vi "Check Data Model.vi"(8 "error in (no error)":errorcluster, 11 "device data model in":refnum<class "ICPCON ET Data Model.lvclass">) -> (0 "error out":errorcluster, 3 "device data model out":refnum<class "ICPCON ET Data Model.lvclass">)   [LabVIEW 2021, in "ICPCON ET Data Model.lvclass"]
doc: "This VI ensures that the data model has at least 65,535 values of every type. This is required for certain modbus function codes."
uses:
  ICPCON ET Data Model.lvclass
  ICPCON ET Data Model.lvclass/ICPCON ET Data Model.ctl
  Type Definitions/Data Model.ctl
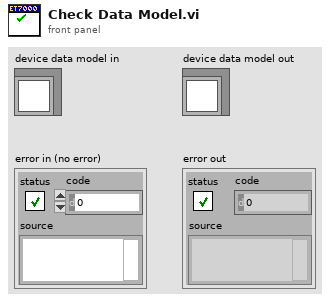
[diagram p1: front panel]
types:
  T1 = typedef "ICPCON ET Data Model.lvclass/Data Model.ctl" = cluster{"UTC":u64, "DI":bool[], "DO":bool[], "IR":u16[], "HR":u16[], "ES":u8}
  T2 = typedef "Device Data Model.lvclass/N channel.ctl" = cluster{"N DI channel":i32, "N DO channel":i32, "N AI channel":i32, "N AO channel":i32}
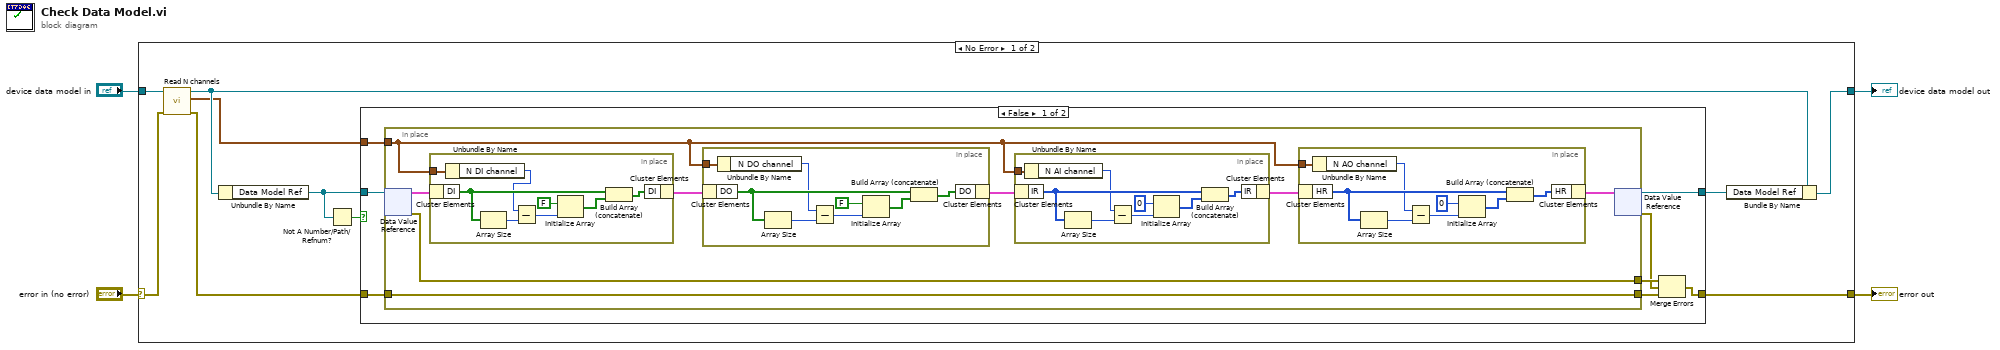
[diagram p0: block diagram]
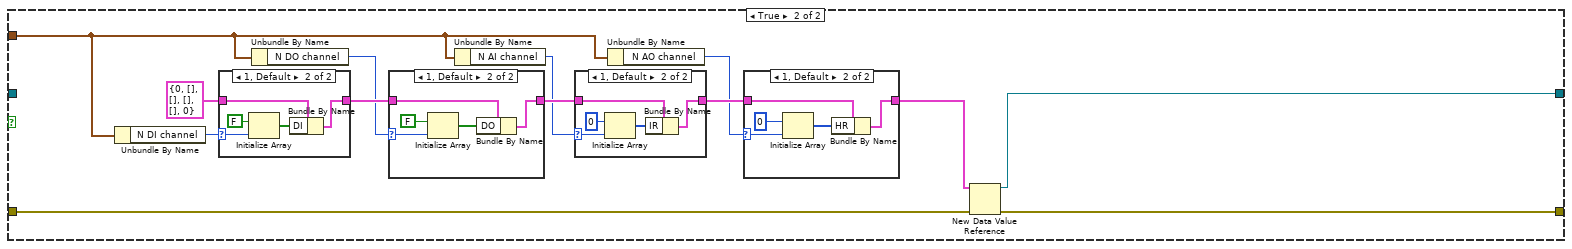
[diagram p2: hidden frame]
diagram:
  n1 = case shown="No Error" "error in (no error)" {
    selector: "error in (no error)" -> [w7 w101]
    tunnel: "device data model in" -> [w9 w100]
    tunnel: [w14 w100] -> w3
    tunnel: [w10 w101] -> w2
    frame No Error {
      n2 = call-dynamic "Read N channels.vi"("error in (no error)"=w7, "device data model in"=w9) -> ("error out"=w6:errorcluster, "N channel"=w5:T2, "device data model out"=w8:refnum<class "ICPCON ET Data Model.lvclass">)  [unwired: 7 in]
      n3 = Unbundle By Name(w8) -> ("Data Model Ref"=w12:refnum<data-value>)
      n4 = Not A Number/Path/Refnum?(number/path/refnum=w12) -> (NaN/Path/Refnum?=w11:bool)
      n5 = case shown="False" w11 {
        tunnel: w6 -> [w22 w75]
        tunnel: w12 -> [w21 _]
        tunnel: [w20 w73] -> w13
        tunnel: [w18 w74] -> w10
        tunnel: w5 -> [w15 w64]
        frame False {
          n6 = in-place {
            in-place-border: w22 -> [w24]
            in-place-border: [w25] -> w19
            in-place-border: [w24] -> w16
            in-place-border: w15 -> [w23]
            n7 = in-place-dvr #1(w21) -> (w30:T1, w25:errorcluster)
            n8 = in-place {
              in-place-border: w23 -> [w56]
              n9 = in-place-cluster #2(w30) -> ("DI"=w59:bool[])
              n10 = Unbundle By Name(w56) -> ("N DI channel"=w55:i32)
              n11 = Array Size(array=w59) -> (size(s)=w62:i32)
              n12 = Subtract(x=w55, y=w62) -> (x-y=w61:i32)
              n13 = Initialize Array(FALSE ("Boolean"), w61) -> (w60:bool[])
              n14 = Build Array (concatenate)(w59, w60) -> (w57:bool[])
              n15 = in-place-cluster #2("DI"=w57) -> (w29:T1)
            }
            n16 = in-place {
              in-place-border: w23 -> [w48]
              n17 = in-place-cluster #3(w29) -> ("DO"=w52:bool[])
              n18 = Unbundle By Name(w48) -> ("N DO channel"=w47:i32)
              n19 = Array Size(array=w52) -> (size(s)=w54:i32)
              n20 = Subtract(x=w47, y=w54) -> (x-y=w50:i32)
              n21 = Initialize Array(FALSE ("Boolean"), w50) -> (w53:bool[])
              n22 = Build Array (concatenate)(w52, w53) -> (w49:bool[])
              n23 = in-place-cluster #3("DO"=w49) -> (w27:T1)
            }
            n24 = in-place {
              in-place-border: w23 -> [w39]
              n25 = in-place-cluster #4(w27) -> ("IR"=w43:u16[])
              n26 = Unbundle By Name(w39) -> ("N AI channel"=w40:i32)
              n27 = Array Size(array=w43) -> (size(s)=w46:i32)
              n28 = Subtract(x=w40, y=w46) -> (x-y=w45:i32)
              n29 = Initialize Array(u16 0, w45) -> (w44:u16[])
              n30 = Build Array (concatenate)(w43, w44) -> (w42:u16[])
              n31 = in-place-cluster #4("IR"=w42) -> (w28:T1)
            }
            n32 = in-place {
              in-place-border: w23 -> [w32]
              n33 = in-place-cluster #5(w28) -> ("HR"=w36:u16[])
              n34 = Unbundle By Name(w32) -> ("N AO channel"=w31:i32)
              n35 = Array Size(array=w36) -> (size(s)=w38:i32)
              n36 = Subtract(x=w31, y=w38) -> (x-y=w35:i32)
              n37 = Initialize Array(u16 0, w35) -> (w37:u16[])
              n38 = Build Array (concatenate)(w36, w37) -> (w34:u16[])
              n39 = in-place-cluster #5("HR"=w34) -> (w26:T1)
            }
            n40 = in-place-dvr #1(w26) -> (w20:refnum<data-value>, w17:errorcluster)
          }
          n41 = Merge Errors(w19, w17, w16) -> (w18:errorcluster)
        }
        frame True {
          n42 = Unbundle By Name(w64) -> ("N DI channel"=w68:i32)
          n43 = case shown="1, Default" w68 {
            selector: w68 -> [_ w83]
            tunnel: T1 {"UTC"=0, "DI"=[], "DO"=[], "IR"=[], "HR"=[], "ES"=0} ("Data Model") -> [w82 w86]
            tunnel: [w82 w84] -> w72
            frame 0 {
            }
            frame 1, Default {
              n44 = Initialize Array(FALSE ("Boolean"), w83) -> (w85:bool[])
              n45 = Bundle By Name(cluster=w86, "DI"=w85) -> (w84:T1)
            }
          }
          n46 = Unbundle By Name(w64) -> ("N DO channel"=w67:i32)
          n47 = case shown="1, Default" w67 {
            selector: w67 -> [_ w78]
            tunnel: w72 -> [w76 w81]
            tunnel: [w76 w79] -> w70
            frame 0 {
            }
            frame 1, Default {
              n48 = Initialize Array(FALSE ("Boolean"), w78) -> (w80:bool[])
              n49 = Bundle By Name(cluster=w81, "DO"=w80) -> (w79:T1)
            }
          }
          n50 = Unbundle By Name(w64) -> ("N AI channel"=w66:i32)
          n51 = case shown="1, Default" w66 {
            selector: w66 -> [_ w96]
            tunnel: w70 -> [w94 w99]
            tunnel: [w94 w97] -> w71
            frame 0 {
            }
            frame 1, Default {
              n52 = Initialize Array(u16 0, w96) -> (w98:u16[])
              n53 = Bundle By Name(cluster=w99, "IR"=w98) -> (w97:T1)
            }
          }
          n54 = Unbundle By Name(w64) -> ("N AO channel"=w65:i32)
          n55 = case shown="1, Default" w65 {
            selector: w65 -> [_ w90]
            tunnel: w71 -> [w88 w93]
            tunnel: [w88 w91] -> w63
            frame 0 {
            }
            frame 1, Default {
              n56 = Initialize Array(u16 0, w90) -> (w92:u16[])
              n57 = Bundle By Name(cluster=w93, "HR"=w92) -> (w91:T1)
            }
          }
          n58 = New Data Value Reference(data value=w63, error in=w75) -> (data value reference=w73:refnum<data-value>, error out=w74:errorcluster)
        }
      }
      n59 = Bundle By Name(cluster=w8, "Data Model Ref"=w13) -> (w14:refnum<class "ICPCON ET Data Model.lvclass">)
    }
    frame Error {
    }
  }
  "error out" <- w2
  "device data model out" <- w3
